vi "SHG Spectra Collection and Trace Generation.vi"(0 "Wavelengths":dbl[](array[numeric]), 1 "Net Phase":dbl[](array[numeric]), 2 "File (SHG Spectra)":path=path "C:/Data/Data", 3 "SLM COM Port":refnum<visa-resource-name>="COM9", 4 "Start":dbl, 5 "Scan range":dbl, 6 "Length":dbl, 7 "Start":dbl, 9 "Increment":dbl, 11 "Parsed formula node reference function":T2, 12 "Slave Mask Calibration":path, 13 "Master Mask Calibration":path) -> (10 "Trace (r=wl, c=d)":dbl[][](array[numeric]), 15 "Deltas":dbl[](array[numeric]))   [LabVIEW 2019]
uses:
  <vilib>/gmath/NI_Gmath.lvlib
panel:
  out "XY Graph":T1(graph)
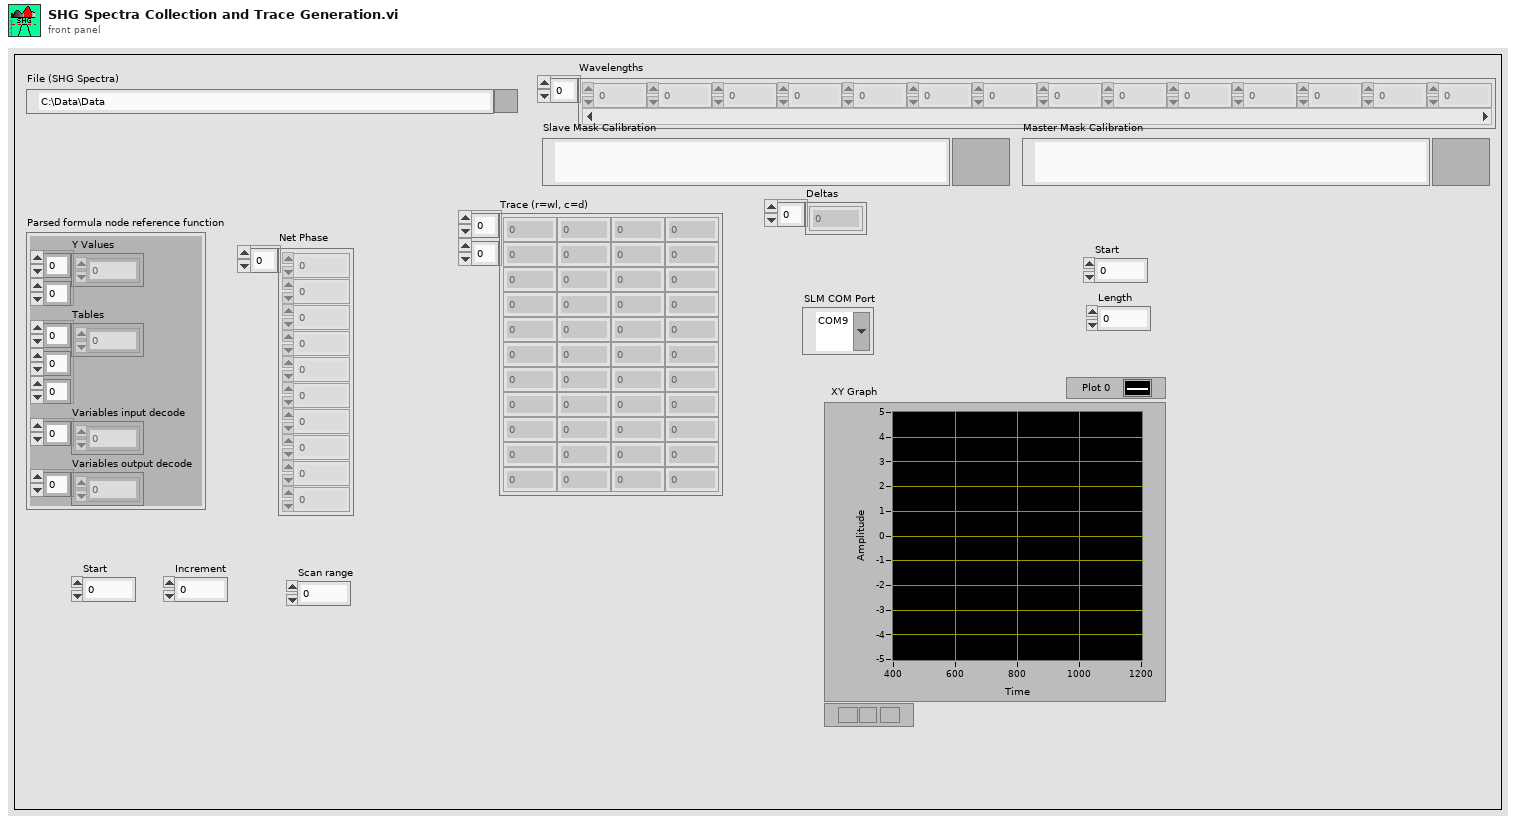
[diagram p1: front panel]
types:
  T1 = cluster{"Wavelengths":dbl[], "FH spectrum":dbl[]}
  T2 = cluster{"Y Values":dbl[][], "Tables":i32[][][], "Variables input decode":i32[], "Variables output decode":i32[]}
  T3 = cluster{cluster{"Wavelengths":dbl[], "Spectrum":dbl[]}[]}
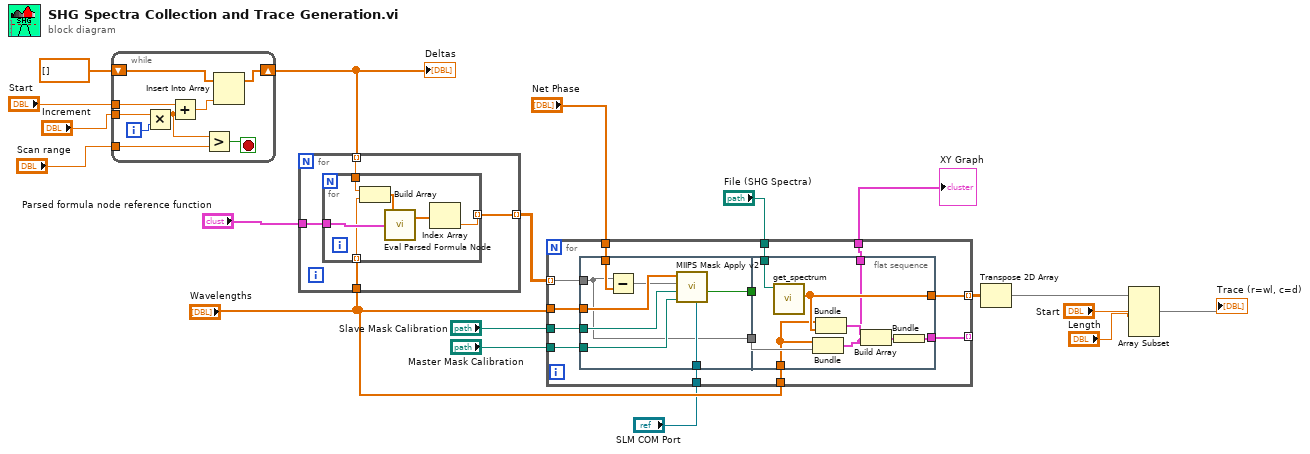
[diagram p0: block diagram]
diagram:
  n1 = while {
    tunnel: "Start" -> [w28]
    tunnel: "Increment" -> [w27]
    tunnel: "Scan range" -> [w24]
    shift-right: [w20] -> w11
    shift-left: dbl[] [] -> [w21]
    i -> [w26]
    stop <- w22 stop-if-true
    n2 = Multiply(x=w27, y=w26) -> (x*y=w23:dbl)
    n3 = Add(x=w28, y=w23) -> (x+y=w25:dbl)
    n4 = Greater?(x=w23, y=w24) -> (0:w22:bool)
    n5 = Insert Into Array(array=w21, new element=w25) -> (w20:dbl[])  [unwired: 1 in]
  }
  "Deltas" <- w11
  n6 = for {
    tunnel: "Parsed formula node reference function" -> [w32]
    tunnel: w11 -> [w31] mode=indexing
    tunnel: "Wavelengths" -> [w30]
    tunnel: [w29] -> w10 mode=indexing
    n7 = for {
      tunnel: w32 -> [w38]
      tunnel: w31 -> [w36]
      tunnel: w30 -> [w35] mode=indexing
      tunnel: [w33] -> w29 mode=indexing
      n8 = Build Array(w36, w35) -> (w37:dbl[])
      n9 = call <vilib>:"Eval Parsed Formula Node.vi"("Parsed Formula Node"=w38, "Input Values"=w37) -> ("Output Values"=w34:dbl[])  [unwired: 1 in, 1 out]
      n10 = Index Array(array=w34) -> (element=w33:dbl)  [unwired: 1 in]
    }
  }
  n11 = for {
    tunnel: "Wavelengths" -> [w51]
    tunnel: "Slave Mask Calibration" -> [w50]
    tunnel: "Master Mask Calibration" -> [w49]
    tunnel: [w48] -> w8 mode=indexing
    tunnel: "Net Phase" -> [w47]
    tunnel: w10 -> [w46] mode=indexing
    tunnel: "File (SHG Spectra)" -> [w45]
    tunnel: "SLM COM Port" -> [w44]
    tunnel: "Wavelengths" -> [w41]
    tunnel: [w40] -> _ mode=indexing
    tunnel: [w39] -> w5
    n12 = flat-sequence {
      tunnel: w51 -> [w59]
      tunnel: w50 -> [w55]
      tunnel: w49 -> [w58]
      tunnel: w47 -> [w57]
      tunnel: w46 -> [w52]
      tunnel: w44 -> [w54]
      tunnel: [w53] -> w43
      tunnel: [w52] -> w42
      tunnel: [w66] -> w48
      tunnel: w45 -> [w67]
      tunnel: w43 -> [_]
      tunnel: w42 -> [w65]
      tunnel: w41 -> [w64]
      tunnel: [w63] -> w40
      tunnel: [w60] -> w39
      frame #0 {
        n13 = Subtract(x=w52, y=w57) -> (x-y=w56:dbl[])
        n14 = call "MIIPS Mask Apply v2.vi"("SLM COM Port"=w54, "Master Mask Calibration"=w58, "Slave Mask Calibration"=w55, "Phase"=w56, "Wavelength"=w59) -> ("Applied"=w53:bool)  [unwired: 4 in, 2 out]
      }
      frame #1 {
        n15 = call "get_spectrum.vi"("File (SHG Spectra)"=w67) -> ("Spectrum"=w66:dbl[])  [unwired: 9 in, 1 out]
        n16 = Bundle("Wavelengths"=w64, w65) -> (w60:cluster{"Wavelengths":dbl[], dbl[]})  [unwired: 1 in]
        n17 = Bundle("Wavelengths"=w64, "Spectrum"=w66) -> (w61:cluster{"Wavelengths":dbl[], "Spectrum":dbl[]})  [unwired: 1 in]
        n18 = Build Array(w61, w60) -> (w62:cluster{"Wavelengths":dbl[], "Spectrum":dbl[]}[])
        n19 = Bundle(w62) -> (w63:T3)  [unwired: 1 in]
      }
    }
  }
  "XY Graph" <- w5
  n20 = Transpose 2D Array(2D array=w8) -> (transposed array=w2:dbl[][])
  n21 = Array Subset(array=w2, index (row)="Start", length (row)="Length") -> (→"Trace (r=wl, c=d)":dbl[][])  [unwired: 2 in]
